vi "UI Events On.vi"(8 "error in (no error)":errorcluster, 10 "UI Events":T1, 11 "Actor_Controller_Template in":refnum<class "Actor_Controller_Template.lvclass">) -> (0 "error out":errorcluster, 3 "Actor_Controller_Template out":refnum<class "Actor_Controller_Template.lvclass">)   [LabVIEW 2020, in "Actor_Controller_Template.lvlib" / "Actor_Controller_Template.lvclass"]
uses:
  Actor_Controller_Template.lvclass
  Actor_UI_Template/UI Event Enum.ctl
  Actor_Controller_Template.lvclass/Actor_Controller_Template.ctl
  Actor_UI_Template/Actor_UI_Template.lvlib
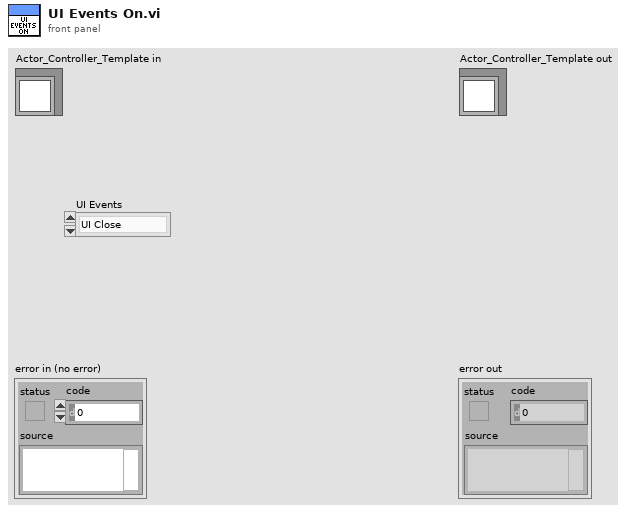
[diagram p1: front panel]
types:
  T1 = typedef "Actor_UI_Template.lvlib/UI Event Enum.ctl" = enum16{"UI Close"}
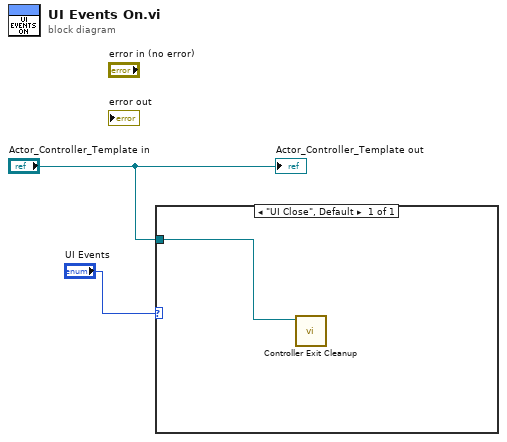
[diagram p0: block diagram]
diagram:
  n1 = case shown="\"UI Close\", Default" "UI Events" {
    tunnel: "Actor_Controller_Template in" -> [w3]
    frame "UI Close", Default {
      n2 = call-dynamic "Controller Exit Cleanup.vi"("Actor_Controller_Template in"=w3) -> ()  [unwired: 9 in, 2 out]
    }
  }
  "Actor_Controller_Template out" <- "Actor_Controller_Template in"
